vi "Operation Parser.vi"(10 "8bit ? 8bit : 4bit (8bit)":bool, 11 "operation":u32) -> (0 "E1? E1: E2 (E1)":bool, 1 "RS":bool, 2 "cmd/data":u8, 3 "command type":enum8{"Write", "Read", "Initialize Entry"}(ring))   [LabVIEW 2017, in "HD44780 FPGA.lvlib"]
uses:
  HD44780 FPGA.lvlib
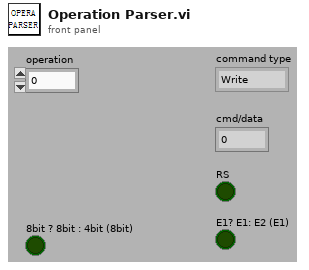
[diagram p1: front panel]
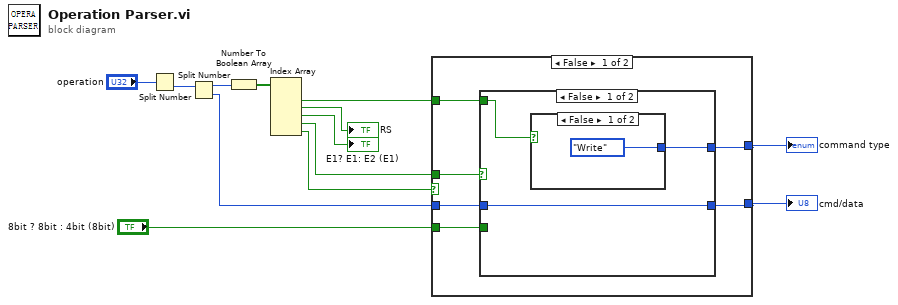
[diagram p0: block diagram]
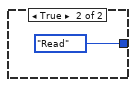
[diagram p2: hidden frame]
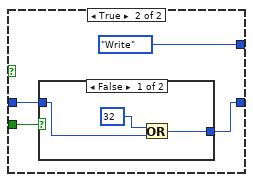
[diagram p3: hidden frame]
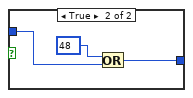
[diagram p4: hidden frame]
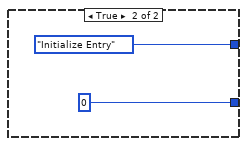
[diagram p5: hidden frame]
diagram:
  n1 = Split Number(x="operation") -> (lo(x)=w8:u16)  [unwired: 1 out]
  n2 = Split Number(x=w8) -> (hi(x)=w13:u8, lo(x)=w4:u8)
  n3 = Number To Boolean Array(number=w13) -> (Boolean array=w12:bool[])
  n4 = Index Array(array=w12) -> (element #1=w7:bool, element #2=→"RS":bool, element #3=→"E1? E1: E2 (E1)":bool, element #4=w6:bool, element #5=w3:bool)  [unwired: 5 in]
  n5 = case shown="False" w3 {
    tunnel: w7 -> [w16 _]
    tunnel: w6 -> [w19 _]
    tunnel: "8bit ? 8bit : 4bit (8bit)" -> [w18 _]
    tunnel: w4 -> [w17 _]
    tunnel: [w15 enum8{"Write", "Read", "Initialize Entry"}."Initialize Entry" ("command type 2")] -> w2
    tunnel: [w14 u8 0] -> w1
    frame False {
      n6 = case shown="False" w19 {
        tunnel: w16 -> [w22 _]
        tunnel: w18 -> [_ w27]
        tunnel: w17 -> [w21 w28]
        tunnel: [w21 w26] -> w14
        tunnel: [w20 enum8{"Write", "Read", "Initialize Entry"}."Write" ("command type 2")] -> w15
        frame False {
          n7 = case shown="False" w22 {
            tunnel: [enum8{"Write", "Read", "Initialize Entry"}."Write" ("command type 2") enum8{"Write", "Read", "Initialize Entry"}."Read" ("command type 2")] -> w20
            frame False {
            }
            frame True {
            }
          }
        }
        frame True {
          n8 = case shown="False" w27 {
            tunnel: [w29 w32] -> w26
            tunnel: w28 -> [w30 w33]
            frame False {
              n9 = Or(x=u8 32, y=w30) -> (x .or. y?=w29:u8)
            }
            frame True {
              n10 = Or(x=u8 48, y=w33) -> (x .or. y?=w32:u8)
            }
          }
        }
      }
    }
    frame True {
    }
  }
  "command type" <- w2
  "cmd/data" <- w1
